vi "ChooseZones.vi"(0 "object in":refnum<class "Team.lvclass">, 2 "Field":refnum<class "Field.lvclass">, 4 "NumberOfAttackers":i32, 5 "error in (no error)":errorcluster) -> (14 "object out":refnum<class "Team.lvclass">, 16 "Zones":refnum<class "Zone.lvclass">[](array[class]), 19 "error out":errorcluster)   [LabVIEW 2023, in "Team.lvclass"]
uses:
  Team.lvclass
  Field_class/Field.lvclass
  Zone_class/Zone.lvclass
  Team.lvclass/Team.ctl
  Zone_class/zones.ctl
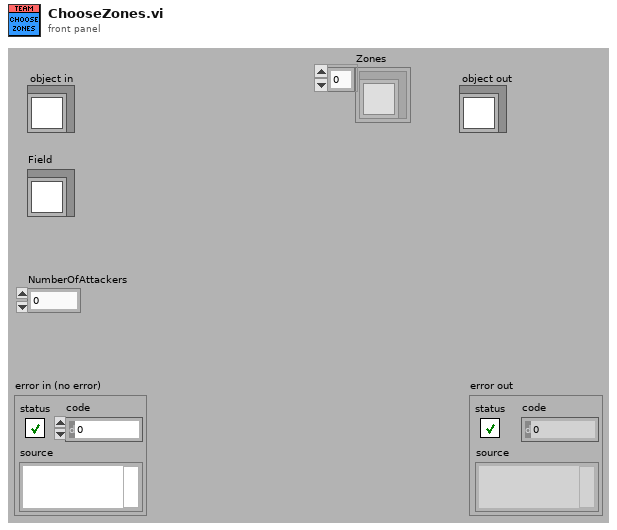
[diagram p1: front panel]
types:
  T1 = typedef "Zone.lvclass/zones.ctl" = enum16{"leftMidField", "rightMidField", "MidField", "leftWing", "rightWing", "LeftSide", "RightSide", "Field", "Size"}
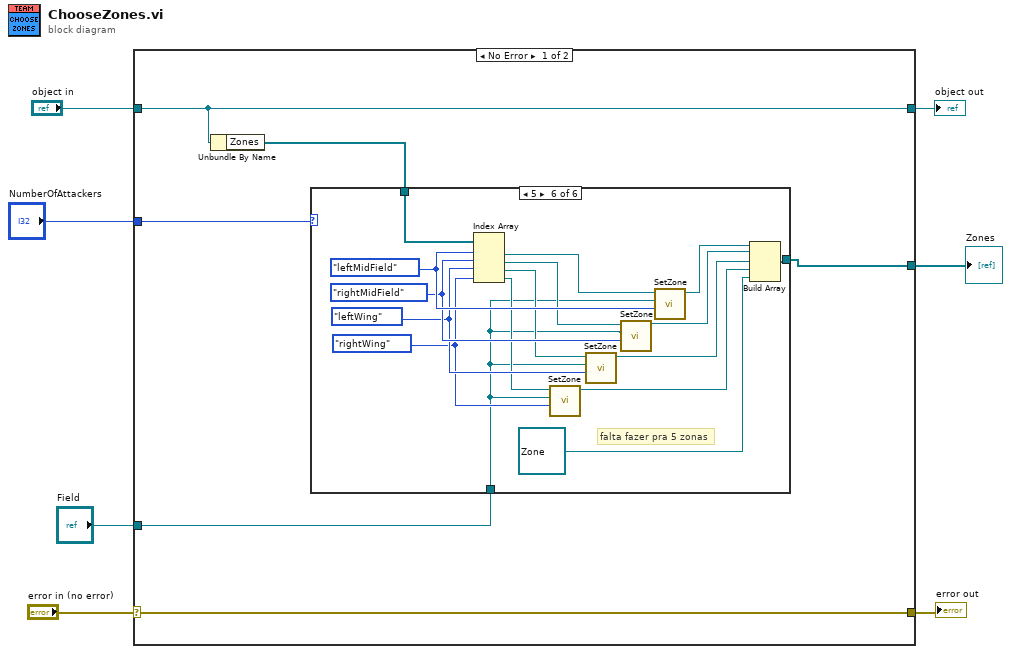
[diagram p0: block diagram]
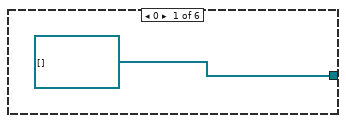
[diagram p2: hidden frame]
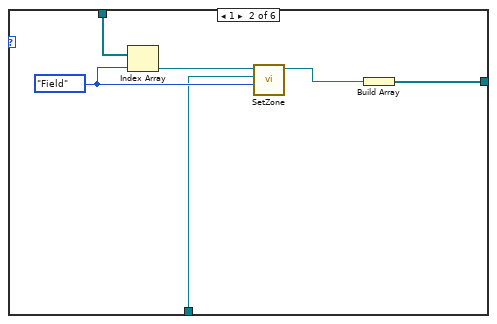
[diagram p3: hidden frame]
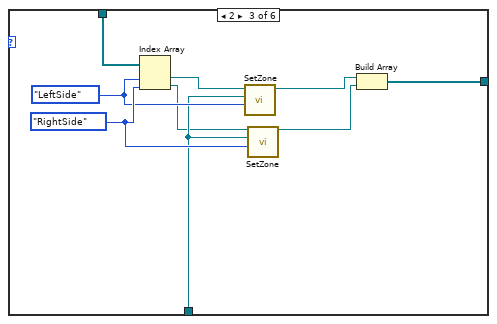
[diagram p4: hidden frame]
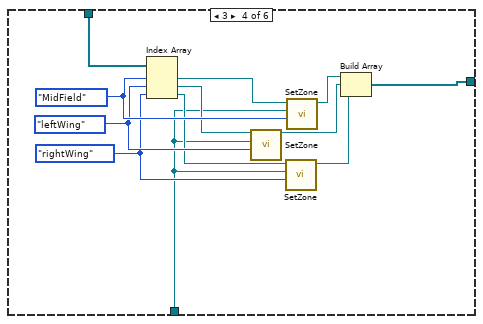
[diagram p5: hidden frame]
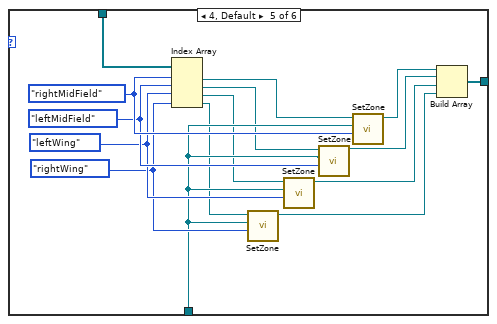
[diagram p6: hidden frame]
diagram:
  n1 = case shown="No Error" "error in (no error)" {
    selector: "error in (no error)" -> [w13 w74]
    tunnel: [w13 w74] -> w6
    tunnel: [w11 w73] -> w4
    tunnel: "object in" -> [w11 w73]
    tunnel: "Field" -> [w12 _]
    tunnel: [w9 _] -> w2
    tunnel: "NumberOfAttackers" -> [w8 _]
    frame No Error {
      n2 = Unbundle By Name(w11) -> ("Zones"=w10:refnum<class "Zone.lvclass">[])
      n3 = case shown="5" w8 {
        tunnel: [refnum<class "Zone.lvclass">[] [] ("Zones") w20 w25 w41 w56 w59] -> w9
        tunnel: w10 -> [_ w16 w21 w33 w47 w60]
        tunnel: w12 -> [_ w15 w24 w30 w45 w58]
        frame 0 {
        }
        frame 1 {
          w18 = zones."Field" ("Enum")
          n4 = Index Array(array=w16, index=w18) -> (element=w17:refnum<class "Zone.lvclass">)
          n5 = call-dynamic "SetZone.vi"("Enum"=w18, "Field"=w15, "object in"=w17) -> ("object out"=w19:refnum<class "Zone.lvclass">)  [unwired: 7 in, 1 out]
          n6 = Build Array(w19) -> (w20:refnum<class "Zone.lvclass">[])
        }
        frame 2 {
          w29 = zones."RightSide" ("Enum")
          w28 = zones."LeftSide" ("Enum")
          n7 = Index Array(array=w21, index #1=w28, index #2=w29) -> (element #1=w23:refnum<class "Zone.lvclass">, element #2=w22:refnum<class "Zone.lvclass">)
          n8 = call-dynamic "SetZone.vi"("Enum"=w28, "Field"=w24, "object in"=w23) -> ("object out"=w27:refnum<class "Zone.lvclass">)  [unwired: 7 in, 1 out]
          n9 = call-dynamic "SetZone.vi"("Enum"=w29, "Field"=w24, "object in"=w22) -> ("object out"=w26:refnum<class "Zone.lvclass">)  [unwired: 7 in, 1 out]
          n10 = Build Array(w27, w26) -> (w25:refnum<class "Zone.lvclass">[])
        }
        frame 3 {
          w38 = zones."rightWing" ("Enum")
          w39 = zones."leftWing" ("Enum")
          w40 = zones."MidField" ("Enum")
          n11 = Index Array(array=w33, index #1=w40, index #2=w39, index #3=w38) -> (element #1=w34:refnum<class "Zone.lvclass">, element #2=w32:refnum<class "Zone.lvclass">, element #3=w31:refnum<class "Zone.lvclass">)
          n12 = call-dynamic "SetZone.vi"("Enum"=w39, "Field"=w30, "object in"=w32) -> ("object out"=w36:refnum<class "Zone.lvclass">)  [unwired: 7 in, 1 out]
          n13 = call-dynamic "SetZone.vi"("Enum"=w38, "Field"=w30, "object in"=w31) -> ("object out"=w35:refnum<class "Zone.lvclass">)  [unwired: 7 in, 1 out]
          n14 = call-dynamic "SetZone.vi"("Enum"=w40, "Field"=w30, "object in"=w34) -> ("object out"=w37:refnum<class "Zone.lvclass">)  [unwired: 7 in, 1 out]
          n15 = Build Array(w37, w36, w35) -> (w41:refnum<class "Zone.lvclass">[])
        }
        frame 4, Default {
          w54 = zones."leftMidField" ("Enum")
          w52 = zones."rightWing" ("Enum")
          w53 = zones."leftWing" ("Enum")
          w55 = zones."rightMidField" ("Enum")
          n16 = Index Array(array=w47, index #1=w55, index #2=w54, index #3=w53, index #4=w52) -> (element #1=w46:refnum<class "Zone.lvclass">, element #2=w42:refnum<class "Zone.lvclass">, element #3=w43:refnum<class "Zone.lvclass">, element #4=w44:refnum<class "Zone.lvclass">)
          n17 = call-dynamic "SetZone.vi"("Enum"=w52, "Field"=w45, "object in"=w44) -> ("object out"=w50:refnum<class "Zone.lvclass">)  [unwired: 7 in, 1 out]
          n18 = call-dynamic "SetZone.vi"("Enum"=w53, "Field"=w45, "object in"=w43) -> ("object out"=w49:refnum<class "Zone.lvclass">)  [unwired: 7 in, 1 out]
          n19 = call-dynamic "SetZone.vi"("Enum"=w54, "Field"=w45, "object in"=w42) -> ("object out"=w48:refnum<class "Zone.lvclass">)  [unwired: 7 in, 1 out]
          n20 = call-dynamic "SetZone.vi"("Enum"=w55, "Field"=w45, "object in"=w46) -> ("object out"=w51:refnum<class "Zone.lvclass">)  [unwired: 7 in, 1 out]
          n21 = Build Array(w51, w48, w49, w50) -> (w56:refnum<class "Zone.lvclass">[])
        }
        frame 5 {
          w71 = zones."rightMidField" ("Enum")
          w69 = zones."rightWing" ("Enum")
          w70 = zones."leftWing" ("Enum")
          w72 = zones."leftMidField" ("Enum")
          # "falta fazer pra 5 zonas"
          n22 = Index Array(array=w60, index #1=w72, index #2=w71, index #3=w70, index #4=w69) -> (element #1=w64:refnum<class "Zone.lvclass">, element #2=w61:refnum<class "Zone.lvclass">, element #3=w62:refnum<class "Zone.lvclass">, element #4=w63:refnum<class "Zone.lvclass">)
          n23 = call-dynamic "SetZone.vi"("Enum"=w69, "Field"=w58, "object in"=w63) -> ("object out"=w67:refnum<class "Zone.lvclass">)  [unwired: 7 in, 1 out]
          n24 = call-dynamic "SetZone.vi"("Enum"=w70, "Field"=w58, "object in"=w62) -> ("object out"=w66:refnum<class "Zone.lvclass">)  [unwired: 7 in, 1 out]
          n25 = call-dynamic "SetZone.vi"("Enum"=w71, "Field"=w58, "object in"=w61) -> ("object out"=w65:refnum<class "Zone.lvclass">)  [unwired: 7 in, 1 out]
          n26 = call-dynamic "SetZone.vi"("Enum"=w72, "Field"=w58, "object in"=w64) -> ("object out"=w68:refnum<class "Zone.lvclass">)  [unwired: 7 in, 1 out]
          n27 = Build Array(w68, w65, w66, w67, refnum<class "Zone.lvclass"> refnum ("element")) -> (w59:refnum<class "Zone.lvclass">[])
        }
      }
    }
    frame Error {
    }
  }
  "error out" <- w6
  "object out" <- w4
  "Zones" <- w2
